vi "DB - [Config].[System].vi"(0 "connection reference":T2, 1 "DB Connection":T3={"Open"=TRUE, "Close"=TRUE}, 3 "[LanguageId]":string="EN", 5 "Date Format (User Defined)":string="%d-%m-%Y", 9 "AND IN (EquipmentIDx,..)":bool, 11 "error in (no error)":errorcluster, 12 "[PlantId]":string="4070", 13 "[SystemId]":string="SRSB-A1", 14 "<Values>":string="'ET-3504 02', 'NI-9211 01','NI-9211 02'") -> (4 "connection reference":T2, 6 "Furnace Details":T1, 10 "Equipment Details (Itemnames)":string[][](array[string]), 15 "SUMMARY":errorcluster)   [LabVIEW 2013]
doc: "-----------------------------------------\n-- Reinehold Systems Solutions Pte Ltd\n-- 2015-01-13 08:46\n------------------------------------------\n \nUSE [SRTRS]\nSELECT\n a.[SerialNo] as [Furnace Serial No]\n ,a.[EquipmentId1] as [Eurotherm]\n ,b.[Model] as [Model]\n ,b.[Description] \n ,b.[SerialNo] as [Equipment Serial No]\n ,b.[EquipmentId]\n ,FORMAT(b.[LastCalibDate], 'yyyy-MM-dd')\n ,FORMAT(b.[NextCalibDate], 'yyyy-MM-dd')\n ,b.[NoticePeriod]\n ,b.[IsCalibRequired]\nFROM [Config].[System] as a\nJOIN [Admin].[Equipment] as b\nON a.[EquipmentId1] = b.[EquipmentId] OR\na.[EquipmentId2] = b.[EquipmentId] OR\na.[EquipmentId3] = b.[EquipmentId] OR\na.[EquipmentId4] = b.[EquipmentId] OR\na.[EquipmentId5] = b.[EquipmentId] OR\na.[EquipmentId6] = b.[EquipmentId] OR\na.[EquipmentId7] = b.[EquipmentId] OR\na.[EquipmentId8] = b.[EquipmentId] \nWHERE \na.[PlantId] = '4070' AND \na.[SystemId] = 'SRSB-A1' AND\na.[Inactive] = '0' AND b.[Inactive] = '0' \nORDER BY b.[Description]"
uses:
  <vilib>/addons/database/Connection.llb/Conn ObjectReference.ctl
  Controls/DB - OpenClose.ctl
  <vilib>/addons/database/Connection.llb/Conn Execute.vi
  <vilib>/addons/database/Recordset.llb/Rec Fetch Recordset Data (R).vi
  <vilib>/addons/database/Recordset.llb/Rec Destroy - Connection.vi
  Controls/Global SRTRS.vi
  <vilib>/addons/database/Connection.llb/DB Tools Open Connec (String).vi
  <vilib>/addons/database/_DB Variant To Data/Database Variant To Data.xnode
  <vilib>/addons/database/NI_Database_API.lvlib
panel:
  in  "Furnace Details":T1={"Furnace Serial No"="A1234A1", "Last Calibration Date"="2012-11-22", "Next Calibration Due Date"="2014-11-22"}
  out "TimeString Error":errorcluster
  out "Close":errorcluster
  in  "DB.Schema.Table \nSRTRS.Config.EquipmentType":string="SRTRS.Config.EquipmentType"
  out "SQL Statement":string
  out "data":string[][](array[string])
  in  "DB.Schema.Table \nSRTRS.Admin.Equipment":string="SRTRS.Admin.Equipment"
  in  "DB.Schema.Table\nSRTRS.Config.System":string="SRTRS.Config.System"
  out "Connection Information":T4={"Connection "="SQL Server 32bit HPEnvy", "Username"="admin", "Password"="admin123"}
  # "2015-01-01 11:19\n[Furnace Serial No]                        [Eurotherm]                                 [Model]                                     [Description]                            [Equipment Serial No]                  [EquipmentId]                           [LastCalibDate]                              [NextCalibDate]                        [NoticePeriod]                          [IsCalibRequired]"
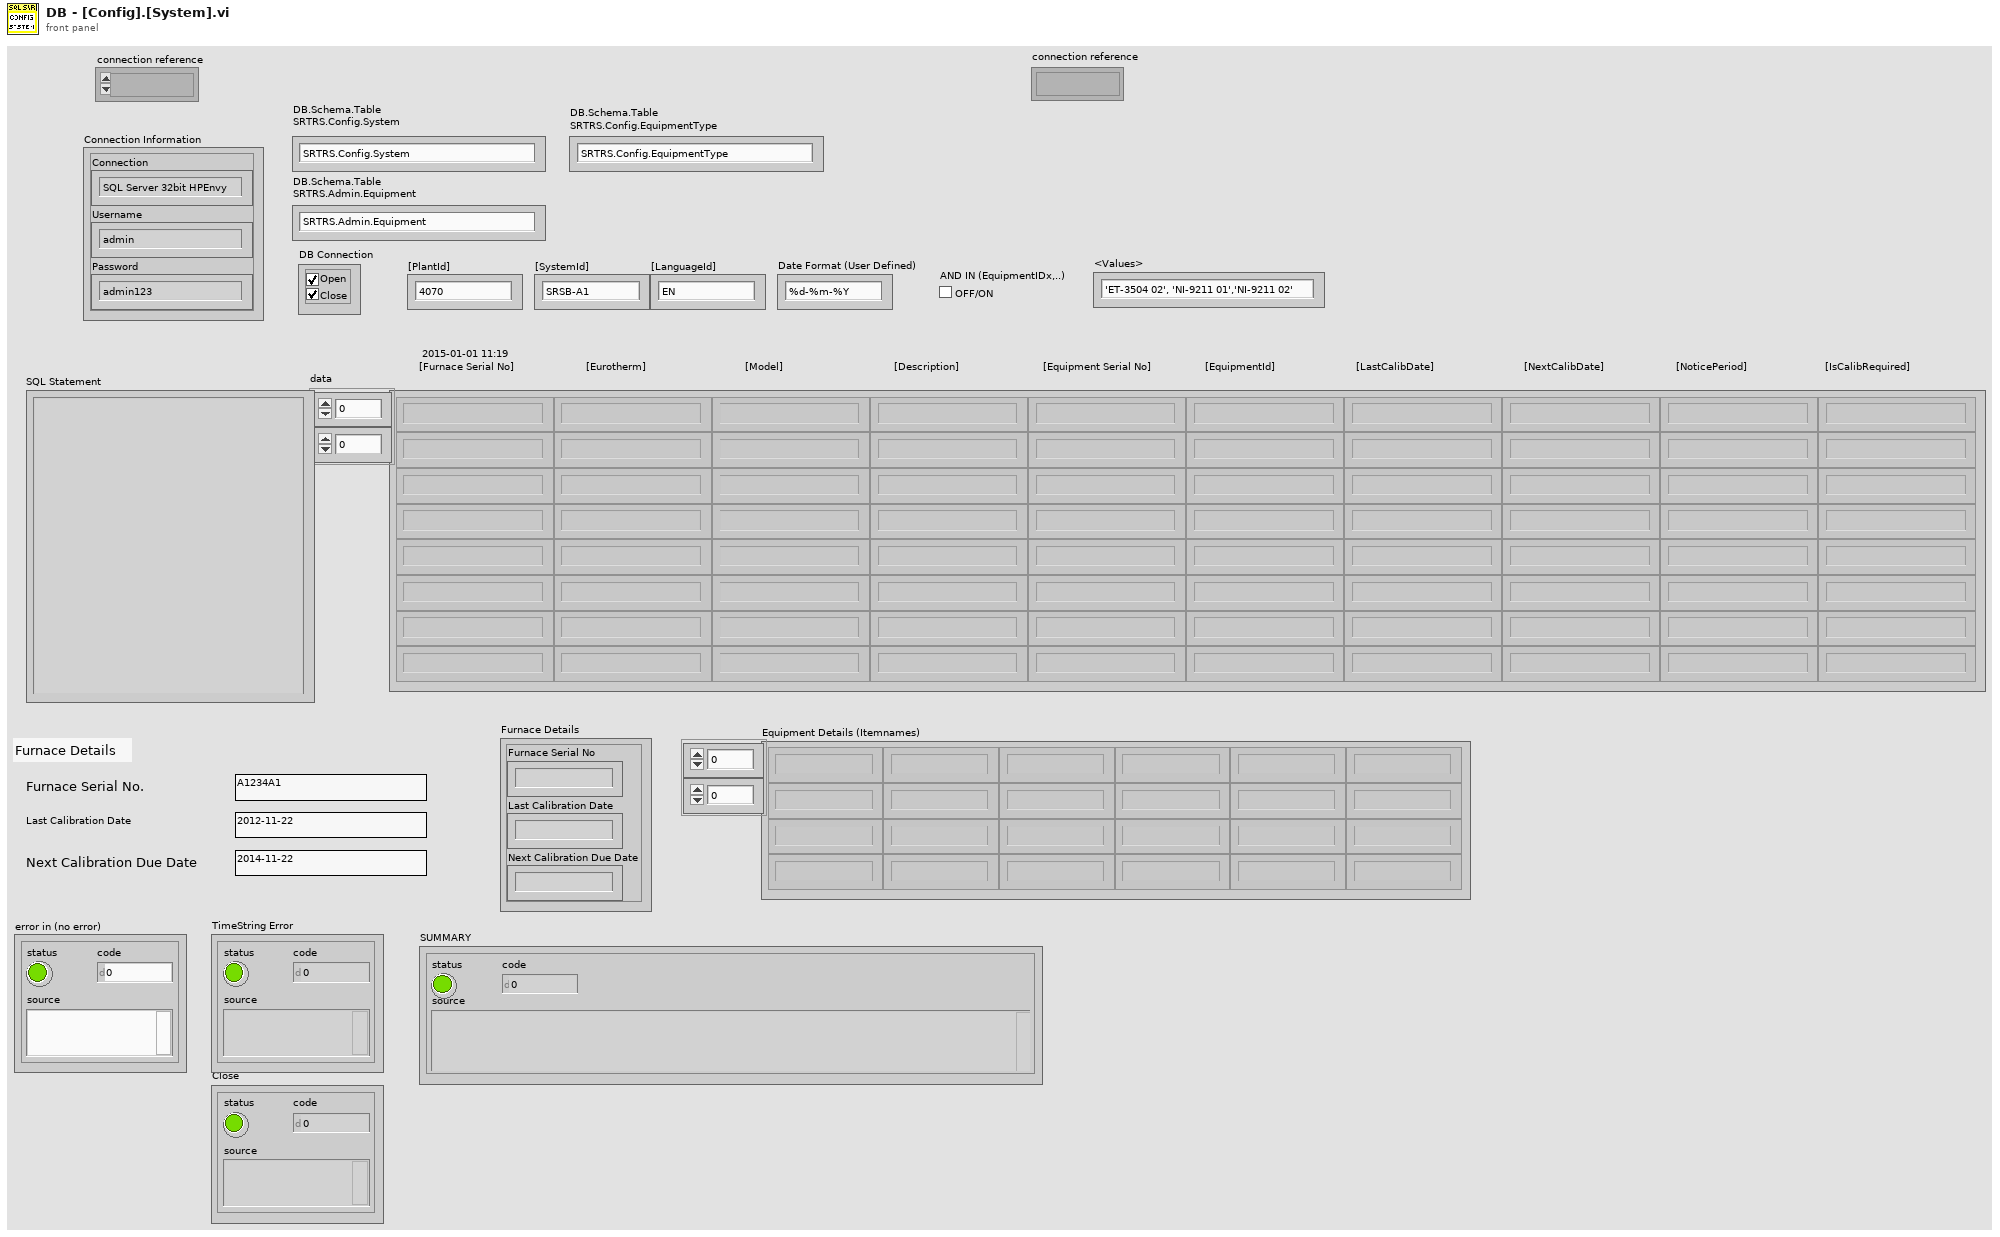
[diagram p1: front panel]
types:
  T1 = cluster{"Furnace Serial No":string, "Last Calibration Date":string, "Next Calibration Due Date":string}
  T2 = typedef "NI_Database_API.lvlib/Conn ObjectReference.ctl" = refnum<k1>
  T3 = typedef "DB - OpenClose.ctl" = cluster{"Open":bool, "Close":bool}
  T4 = cluster{"Connection ":string, "Username":string, "Password":string}
  T5 = typedef "Enum - InteractiveMode-SubVIMode.ctl" = enum16{"Interactive", "subVI Mode"}
  T6 = typedef "DB - DB.Schema.Table.ctl" = cluster{"DB":string, "Schema":string, "Table":string}
  T7 = typedef "Connection Information Cluster.ctl" = cluster{"Connection ":string, "Username":string, "Password":string}
  T8 = typedef "NI_Database_API.lvlib/Rec ObjectReference.ctl" = refnum<k1>
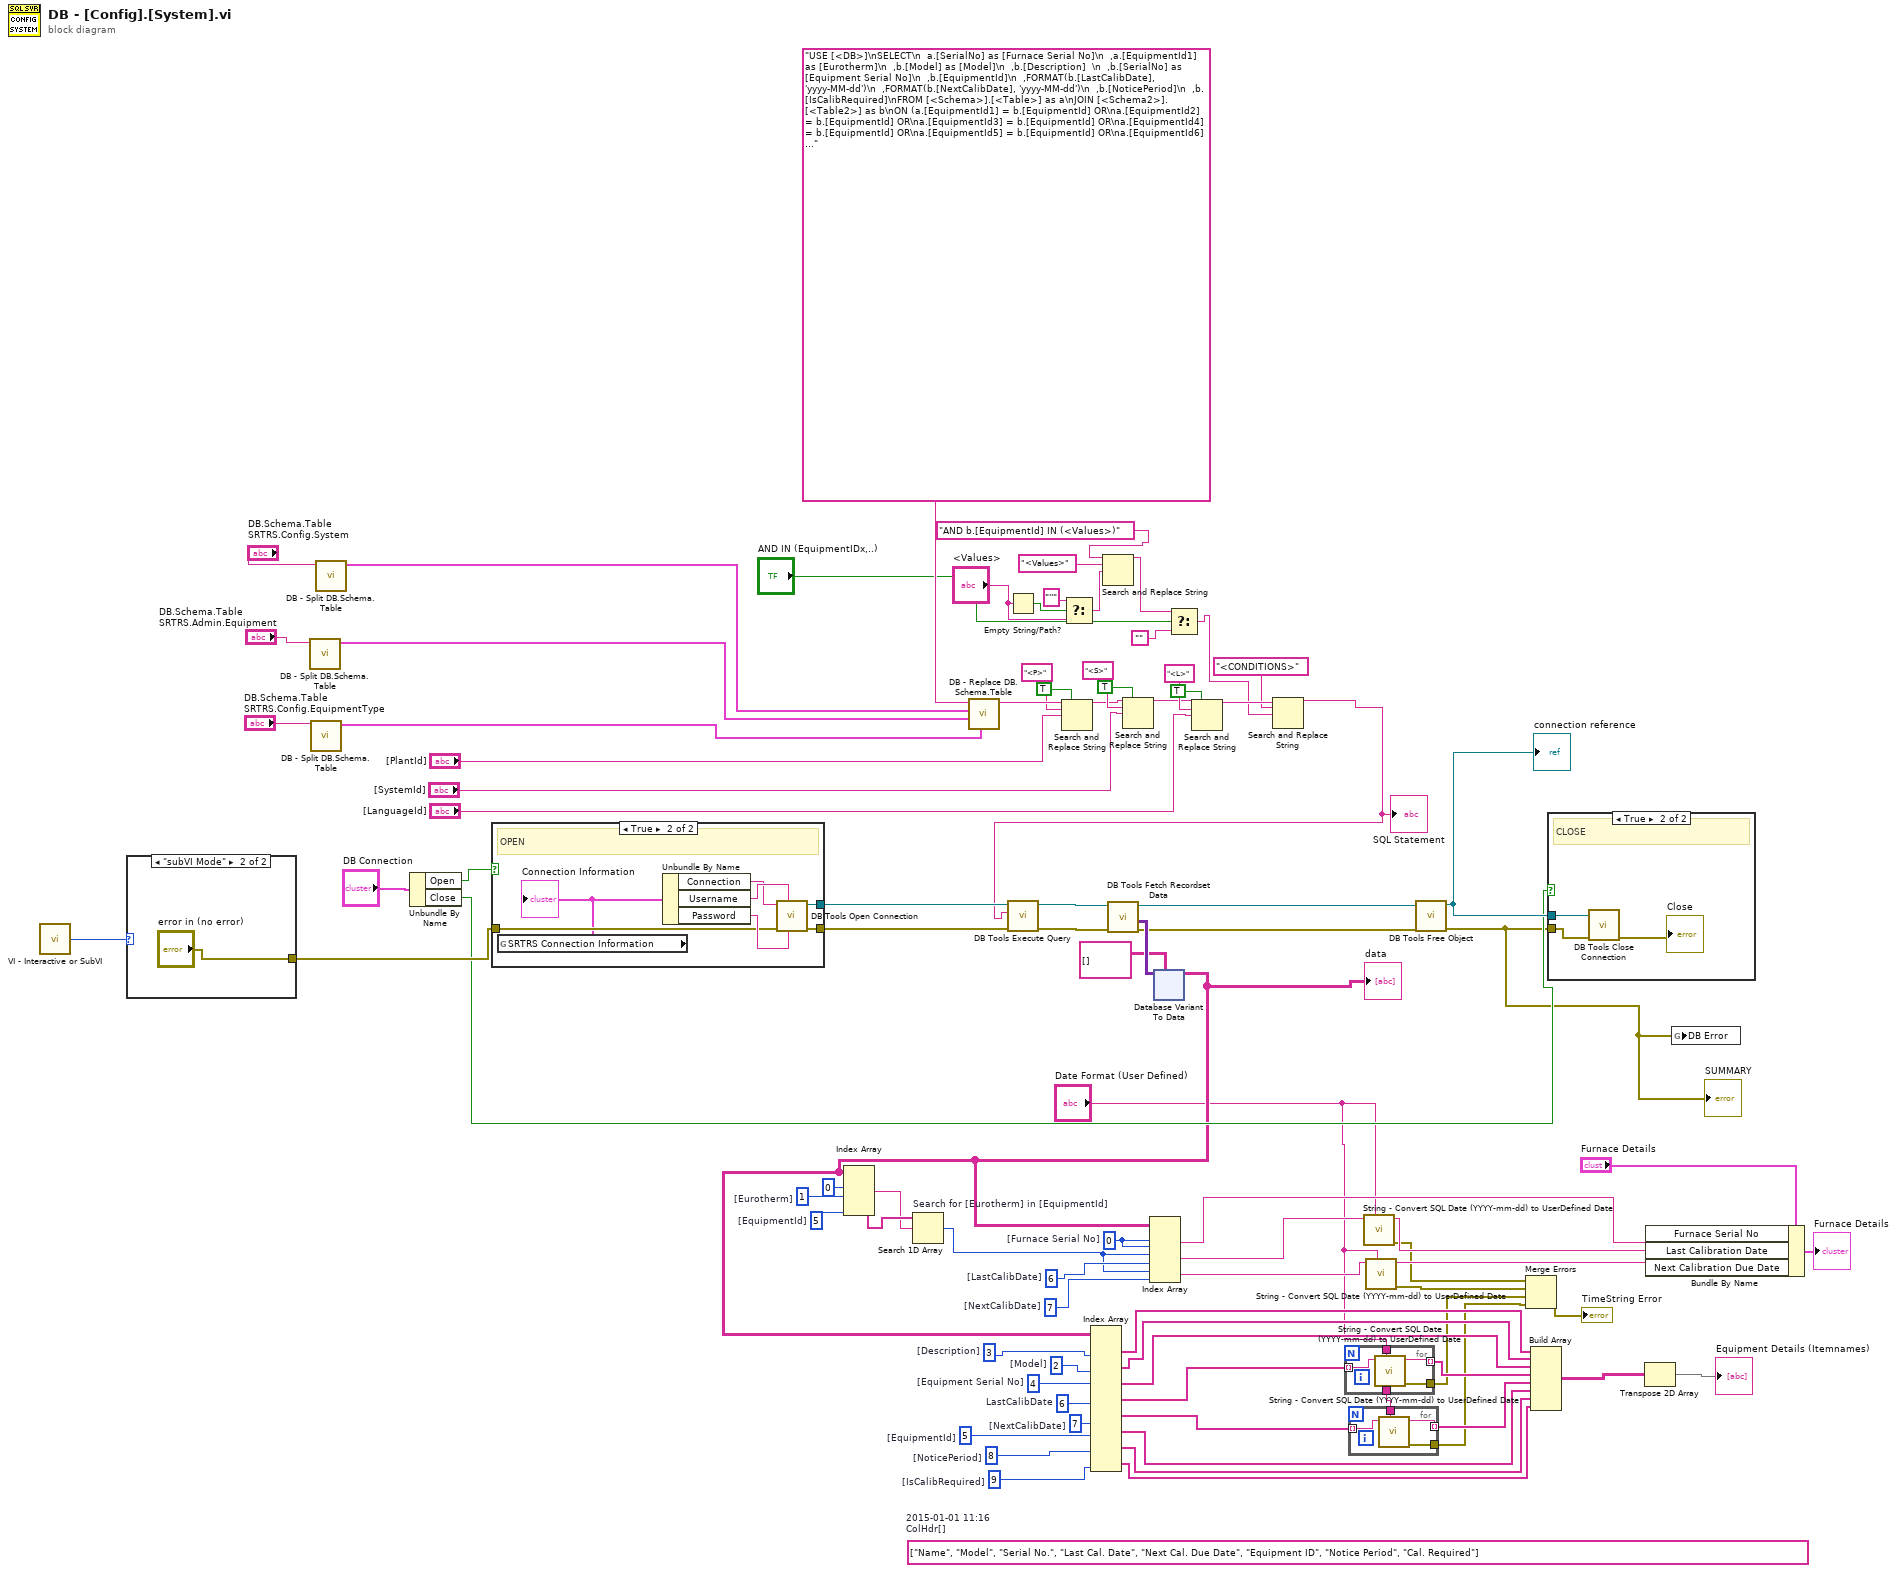
[diagram p0: block diagram]
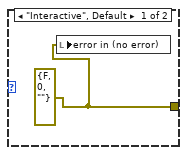
[diagram p3: hidden frame]
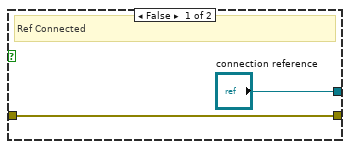
[diagram p4: hidden frame]
diagram:
  w19 = 9  # [IsCalibRequired]
  (unwired) string[] ["Name", "Model", "Serial No.", "Last Cal. Date", "Next Cal. Due Date", "Equipment ID", "Notice Period", "Cal. Required"]  # 2015-01-01 11:16 ColHdr[]
  w40 = 8  # [NoticePeriod]
  w41 = 5  # [EquipmentId]
  w42 = 3  # [Description]
  w45 = 7  # [NextCalibDate]
  w46 = 6  # LastCalibDate
  w47 = 4  # [Equipment Serial No]
  w48 = 2  # [Model]
  w49 = 0  # [Furnace Serial No]
  w50 = 7  # [NextCalibDate]
  w52 = 6  # [LastCalibDate]
  w54 = 1  # [Eurotherm]
  w57 = 5  # [EquipmentId]
  n1 = call "VI - Interactive or SubVI.vi"() -> ("Mode"=w89:T5)  [unwired: 5 in]
  n2 = case shown="\"subVI Mode\"" w89 {
    tunnel: [w92 "error in (no error)"] -> w88
    frame "Interactive", Default {
      w92 = errorcluster {"status"=FALSE, "code"=0, "source"=""} ("error in (no error)")
      n3 = local write "error in (no error)"(w92) -> ()
    }
    frame "subVI Mode" {
    }
  }
  n4 = call "DB - Split DB.Schema.Table.vi"("DB.Schema.Table"="DB.Schema.Table \nSRTRS.Admin.Equipment") -> ("DB.Schema.Table"=w70:T6)  [unwired: 10 in]
  n5 = call "DB - Split DB.Schema.Table.vi"("DB.Schema.Table"="DB.Schema.Table \nSRTRS.Config.EquipmentType") -> ("DB.Schema.Table"=w68:T6)  [unwired: 10 in]
  n6 = call "DB - Split DB.Schema.Table.vi"("DB.Schema.Table"="DB.Schema.Table\nSRTRS.Config.System") -> ("DB.Schema.Table"=w75:T6)  [unwired: 10 in]
  n7 = Unbundle By Name("DB Connection") -> ("Open"=w90:bool, "Close"=w78:bool)
  n8 = case shown="True" w90 {
    tunnel: ["connection reference" w99] -> w81
    tunnel: w88 -> [w94 w98]
    tunnel: [w94 w97] -> w80
    frame False {
      # "Ref Connected"
    }
    frame True {
      # "OPEN"
      n9 = global read "Global SRTRS.vi" "SRTRS Connection Information"() -> (w96:T7)
      "Connection Information" <- w96
      n10 = Unbundle By Name(w96) -> ("Connection"=w101:string, "Username"=w102:string, "Password"=w100:string)
      n11 = call-poly <vilib>:"DB Tools Open Connection.vi"("password"=w100, "userID"=w102, "error in (no error)"=w98, "connection information"=w101) -> ("error out"=w97:errorcluster, "connection reference"=w99:T2)  [unwired: 4 in]
    }
  }
  n12 = call "DB - Replace DB.Schema.Table.vi"("DB.Schema.Table 3"=w68, "DB.Schema.Table 2"=w70, "DB.Schema.Table"=w75, "string in"="USE [<DB>]\nSELECT\n  a.[SerialNo] as [Furnace Serial No]\n  ,a.[EquipmentId1] as [Eurotherm]\n  ,b.[Model] as [Model]\n  ,b.[Description]  \n  ,b.[SerialNo] as [Equipment Serial No]\n  ,b.[EquipmentId]\n  ,FORMAT(b.[LastCalibDate], 'yyyy-MM-dd')\n  ,FORMAT(b.[NextCalibDate], 'yyyy-MM-dd')\n  ,b.[NoticePeriod]\n  ,b.[IsCalibRequired]\nFROM [<Schema>].[<Table>] as a\nJOIN [<Schema2>].[<Table2>] as b\nON (a.[EquipmentId1] = b.[EquipmentId] OR\na.[EquipmentId2] = b.[EquipmentId] OR\na.[EquipmentId3] = b.[EquipmentId] OR\na.[EquipmentId4] = b.[EquipmentId] OR\na.[EquipmentId5] = b.[EquipmentId] OR\na.[EquipmentId6] = b.[EquipmentId] OR\na.[EquipmentId7] = b.[EquipmentId] OR\na.[EquipmentId8] = b.[EquipmentId] )\n\n<CONDITIONS>\n\nWHERE \na.[PlantId] = '<P>' AND \na.[SystemId] = '<S>' AND\na.[Inactive] = '0' AND b.[Inactive] = '0' \nORDER BY b.[Description] ") -> ("string out"=w73:string)  [unwired: 6 in, 1 out]
  n13 = Empty String/Path?(string/path="<Values>") -> (empty?=w4:bool)
  n14 = Search and Replace String(replace all?=TRUE ("replace all? (F)"), input string=w73, search string="<P>", replace string="[PlantId]") -> (result string=w60:string)  [unwired: 4 in, 3 out]
  n15 = Select(t="''", s=w4, f="<Values>") -> (s? t:f=w1:string)
  n16 = Search and Replace String(input string="AND b.[EquipmentId] IN (<Values>)" ("search string"), search string="<Values>", replace string=w1) -> (result string=w5:string)  [unwired: 5 in, 3 out]
  n17 = Search and Replace String(replace all?=TRUE ("replace all? (F)"), input string=w60, search string="<S>", replace string="[SystemId]") -> (result string=w59:string)  [unwired: 4 in, 3 out]
  n18 = Select(t=w5, s="AND IN (EquipmentIDx,..)", f="") -> (s? t:f=w9:string)
  n19 = Search and Replace String(replace all?=TRUE ("replace all? (F)"), input string=w59, search string="<L>", replace string="[LanguageId]") -> (result string=w12:string)  [unwired: 4 in, 3 out]
  n20 = Search and Replace String(input string=w12, search string="<CONDITIONS>", replace string=w9) -> (result string=w11:string)  [unwired: 5 in, 3 out]
  "SQL Statement" <- w11
  n21 = call-poly <vilib>:"DB Tools Execute Query.vi"("error in (no error)"=w80, "SQL query"=w11, "connection reference"=w81) -> ("error out"=w87:errorcluster, "recordset reference"=w86:T8)  [unwired: 5 in]
  n22 = call-poly <vilib>:"DB Tools Fetch Recordset Data.vi"("error in (no error)"=w87, "recordset reference"=w86) -> ("error out"=w82:errorcluster, "recordset data"=w85:variant[][], "recordset reference out"=w83:T8)  [unwired: 3 in]
  n23 = xnode "Database Variant To Data"("database variant"=w85, "type"=string[][] []) -> ("data"=w17:string[][])  [unwired: 1 in, 1 out]
  "data" <- w17
  n24 = Index Array(array=w17, index (row) #1=0, index (col) #1=w54, index (col) #2=w57) -> (element #1=w55:string, element #2=w56:string[])  [unwired: 1 in]
  n25 = Search 1D Array "Search for [Eurotherm] in [EquipmentId]"(1D array=w56, element=w55) -> (index of element=w51:i32)  [unwired: 1 in]
  n26 = Index Array(array=w17, index (col) #1=w42, index (col) #2=w48, index (col) #3=w47, index (col) #4=w46, index (col) #5=w45, index (col) #6=w41, index (col) #7=w40, index (col) #8=w19) -> (element #1=w26:string[], element #2=w25:string[], element #3=w24:string[], element #4=w32:string[], element #5=w28:string[], element #6=w29:string[], element #7=w30:string[], element #8=w18:string[])  [unwired: 8 in]
  n27 = Index Array(array=w17, index (row) #1=w49, index (col) #1=w49, index (row) #2=w51, index (col) #2=w52, index (row) #3=w51, index (col) #3=w50) -> (element #1=w23:string, element #2=w39:string, element #3=w37:string)
  n28 = for {
    tunnel: w32 -> [w106] mode=indexing
    tunnel: "Date Format (User Defined)" -> [w104]
    tunnel: [w105] -> w31 mode=indexing
    tunnel: [w104] -> w22
    tunnel: [w103] -> w21
    n29 = call "String - Convert SQL Date (YYYY-mm-dd) to UserDefined Date.vi"("Date Format (UserDefined)"=w104, "YYYY-mm-dd"=w106) -> ("error out"=w103:errorcluster, "Date String (UserDefined)"=w105:string)  [unwired: 8 in]
  }
  n30 = for {
    tunnel: w28 -> [w110] mode=indexing
    tunnel: w22 -> [w109]
    tunnel: [w108] -> w27 mode=indexing
    tunnel: [w107] -> w20
    n31 = call "String - Convert SQL Date (YYYY-mm-dd) to UserDefined Date.vi"("Date Format (UserDefined)"=w109, "YYYY-mm-dd"=w110) -> ("error out"=w107:errorcluster, "Date String (UserDefined)"=w108:string)  [unwired: 8 in]
  }
  n32 = call "String - Convert SQL Date (YYYY-mm-dd) to UserDefined Date.vi"("Date Format (UserDefined)"="Date Format (User Defined)", "YYYY-mm-dd"=w39) -> ("error out"=w35:errorcluster, "Date String (UserDefined)"=w38:string)  [unwired: 8 in]
  n33 = call "String - Convert SQL Date (YYYY-mm-dd) to UserDefined Date.vi"("Date Format (UserDefined)"="Date Format (User Defined)", "YYYY-mm-dd"=w37) -> ("error out"=w34:errorcluster, "Date String (UserDefined)"=w36:string)  [unwired: 8 in]
  n34 = call-poly <vilib>:"DB Tools Free Object.vi"("error in (no error)"=w82, "recordset reference"=w83) -> ("error out"=w65:errorcluster, "connection reference"=w79:T2)  [unwired: 8 in]
  "SUMMARY" <- w65
  "connection reference" <- w79
  n35 = Merge Errors(w35, w34, w21, w20) -> (→"TimeString Error":errorcluster)
  n36 = Build Array(w26, w25, w24, w31, w27, w29, w30, w18) -> (w44:string[][])
  n37 = case shown="True" w78 {
    tunnel: w79 -> [_ w113]
    tunnel: w65 -> [_ w112]
    frame False {
      # "Ref Connected"
    }
    frame True {
      # "CLOSE"
      n38 = call <vilib>:"DB Tools Close Connection.vi"("error in (no error)"=w112, "connection reference"=w113) -> ("error out"=→"Close":errorcluster)  [unwired: 5 in]
    }
  }
  n39 = Transpose 2D Array(2D array=w44) -> (transposed array=→"Equipment Details (Itemnames)":string[][])
  n40 = Bundle By Name(cluster="Furnace Details", "Furnace Serial No"=w23, "Last Calibration Date"=w38, "Next Calibration Due Date"=w36) -> (→"Furnace Details":T1)
  n41 = global write "Global SRTRS.vi" "DB Error"(w65) -> ()
